vi "db_data_input_b2g_t1_cod_conc.vi"() -> ()   [LabVIEW 2011]
uses:
  <vilib>/Platform/TimedLoop/XDataNode/timing_clust.ctl
  <vilib>/Platform/TimedLoop/XDataNode/nitl_modes.ctl
  <vilib>/Platform/TimedLoop/XDataNode/wakeup.ctl
  <vilib>/addons/database/Connection.llb/DB Tools Open Connec (Path).vi
  <vilib>/Platform/TimedLoop/XDataNode/XDataNode.xnode
  <vilib>/addons/database/_DB Variant To Data/Database Variant To Data.xnode
  <vilib>/Platform/TimedLoop/XDataNode/XDNodeRunTimeDep.lvlib
  <vilib>/addons/database/NI_Database_API.lvlib
panel:
  in  "send data":bool
  in  "COD concentration [mg/l]":u32
  in  "Sampling Timestamp":timestamp format="%<%X\n%x>T"
  in  "Reload":bool
  out "B2G_T1_COD_conc":string[][](table)
  in  "stop":bool
  # "Write COD data of Tank 1 \nto the database"
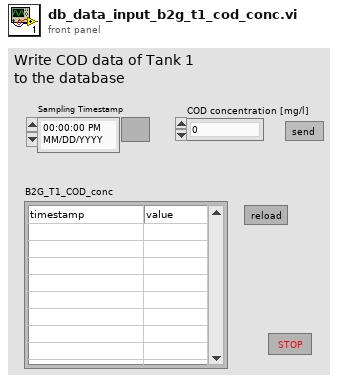
[diagram p1: front panel]
types:
  T1 = typedef "NI_Database_API.lvlib/Conn ObjectReference.ctl" = refnum<k1>
  T2 = typedef "XDNodeRunTimeDep.lvlib/timing_clust.ctl" = cluster{"Expected End [f-1]":u64, "Actual End [f-1]":u64, "Finished Late? [f-1]":bool, "Expected End [i-1]":u64, "Actual End [i-1]":u64, "Finished Late? [i-1]":bool, "Expected Start [i]":u64, "Actual Start [i]":u64, "Expected Start [f]":u64, "Actual Start [f]":u64, "Source Name":string, "Structure Name":string, "Period":i64, "Deadline":i64, "Offset":i64, "Start":i64, "Priority":i32, "Timeout":i32, "Mode":T3, "Wakeup Reason":T4, "Error":errorcluster, "Source Type":string, "Secondary Source Type":string, "Global End Time":u64, "Global Start Time":u64, "Frame Duration":u64, "Iteration Duration":u64, "Assigned CPU":i32, "I/O Scan Engine Mode":u32}
  T3 = typedef "XDNodeRunTimeDep.lvlib/nitl_modes.ctl" = enum32{"No Change", "Process missed periods, maintain original phase", "Discard missed periods, maintain original phase", "Process missed periods, ignore original phase", "Discard missed periods, ignore original phase"}
  T4 = typedef "XDNodeRunTimeDep.lvlib/wakeup.ctl" = enum32{"Normal", "Aborted", "Asynchronous wakeup", "Timing source error", "Timed loop error", "Timeout"}
  T5 = cluster{"Sampling Timestamp":timestamp, "COD concentration [mg/l]":u32}
  T6 = enum32{"invalid app kind", "Development System", "Run Time System", "Student Edition", "Embedded LabVIEW", "Evaluation", "Custom"}
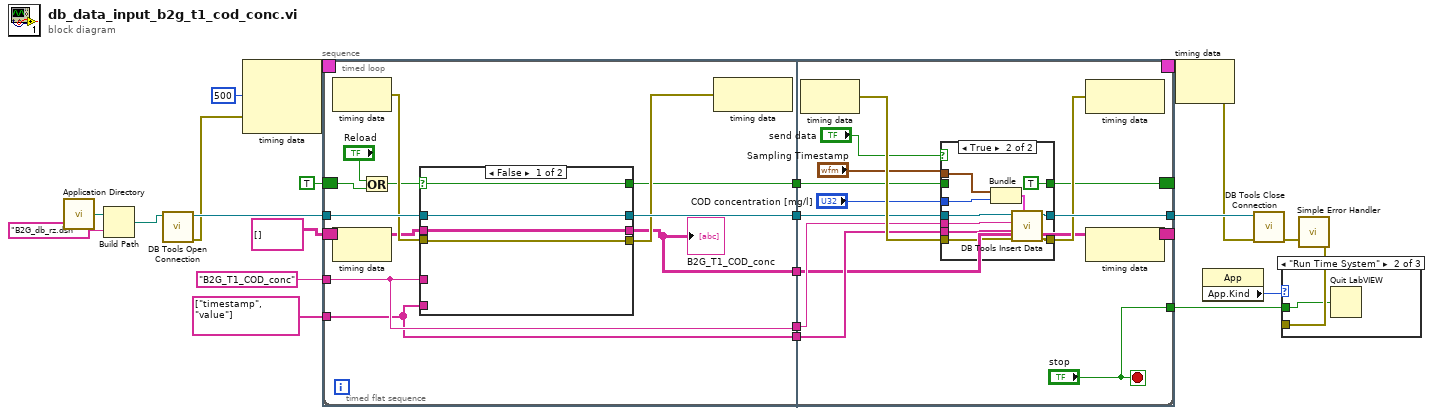
[diagram p0: block diagram]
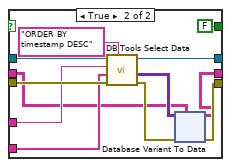
[diagram p4: hidden frame]
diagram:
  n1 = call <vilib>:"Application Directory.vi"() -> ("Application Directory"=w3:path)
  n2 = Build Path(base path=w3, name or relative path="B2G_db_rz.dsn" ("Name of ini file 2")) -> (appended path=w1:path)
  n3 = call-poly <vilib>:"DB Tools Open Connection.vi"("connection information"=w1) -> ("error out"=w13:errorcluster, "connection reference"=w15:T1)  [unwired: 7 in]
  n4 = node-c288(i64 500 ("Period"), w13) -> (w18:T2)  [unwired: 1 in]
  n5 = timed-loop {
    timing: w18 -> [_]
    timing-out: [_] -> w17
    tunnel: w15 -> [w27]
    tunnel: [w26] -> w14
    shift-right: [w25] -> _
    shift-left: TRUE -> [w24]
    tunnel: "B2G_T1_COD_conc" ("table") -> [w23]
    tunnel: string[] ["timestamp", "value"] ("columns") -> [w22]
    tunnel: [w21] -> w7
    shift-right: [w20] -> _
    shift-left: string[][] [] ("data") -> [w19]
    stop <- "stop" stop-if-true
    n6 = timed-sequence {
      timing: _ -> [_]
      timing-out: _ -> [_]
      tunnel: w27 -> [w41]
      tunnel: [w40] -> w26
      tunnel: [w39] -> w25
      tunnel: w24 -> [w38]
      tunnel: w23 -> [w37]
      tunnel: w22 -> [w36]
      tunnel: [w31] -> w21
      tunnel: [w29] -> w20
      tunnel: w19 -> [w28]
      n7 = timed-flat-sequence {
        tunnel: w41 -> [w53]
        tunnel: [w51] -> w35
        tunnel: [w49] -> w34
        tunnel: w38 -> [w48]
        tunnel: w37 -> [w45]
        tunnel: w36 -> [w44]
        tunnel: [w45] -> w33
        tunnel: [w44] -> w32
        tunnel: [w42] -> w30
        tunnel: w28 -> [w46]
        tunnel: [w131] -> w40
        tunnel: w35 -> [w128]
        tunnel: w34 -> [w121]
        tunnel: [w122] -> w39
        tunnel: w33 -> [w127]
        tunnel: w32 -> [w126]
        tunnel: ["stop"] -> w31
        tunnel: w30 -> [w119]
        tunnel: [w119] -> w29
        frame #0 {
          n8 = node-c288() -> (w52:errorcluster)  [unwired: 1 in]
          n9 = Or(x="Reload", y=w48) -> (x .or. y?=w43:bool)
          n10 = case shown="False" w43 {
            selector: w43 -> [w55 _]
            tunnel: w53 -> [w57 w69]
            tunnel: w52 -> [w56 w68]
            tunnel: [w57 w67] -> w51
            tunnel: [w56 w64] -> w50
            tunnel: [w54 w63] -> w42
            tunnel: [w55 FALSE] -> w49
            tunnel: w46 -> [w54 w58]
            tunnel: w45 -> [_ w61]
            tunnel: w44 -> [_ w60]
            frame False {
            }
            frame True {
              n11 = call <vilib>:"DB Tools Select Data.vi"("condition"="ORDER BY timestamp DESC", "error in (no error)"=w68, "columns"=w60, "table"=w61, "connection reference"=w69) -> ("error out"=w65:errorcluster, "data"=w66:variant[][], "connection reference out"=w67:T1)  [unwired: 1 in]
              n12 = xnode "Database Variant To Data"("database variant"=w66, "error in"=w65, "type"=w58) -> ("data"=w63:string[][], "error out"=w64:errorcluster)
            }
          }
          "B2G_T1_COD_conc" <- w42
          n13 = node-c288(w50) -> ()  [unwired: 1 out]
        }
        frame #1 {
          n14 = node-c288() -> (w130:errorcluster)  [unwired: 1 in]
          n15 = case shown="True" "send data" {
            tunnel: [w133 w144] -> w131
            tunnel: w130 -> [w132 w143]
            tunnel: [w132 w142] -> w129
            tunnel: w128 -> [w133 w141]
            tunnel: w127 -> [_ w140]
            tunnel: w126 -> [_ w139]
            tunnel: "Sampling Timestamp" -> [_ w138]
            tunnel: "COD concentration [mg/l]" -> [_ w137]
            tunnel: [w134 TRUE] -> w122
            tunnel: w121 -> [w134 _]
            frame False {
            }
            frame True {
              n16 = Bundle("Sampling Timestamp"=w138, "COD concentration [mg/l]"=w137) -> (w136:T5)  [unwired: 1 in]
              n17 = call <vilib>:"DB Tools Insert Data.vi"("data"=w136, "error in (no error)"=w143, "columns"=w139, "table"=w140, "connection reference"=w141) -> ("error out"=w142:errorcluster, "connection reference out"=w144:T1)  [unwired: 5 in]
            }
          }
          n18 = node-c288(w129) -> ()  [unwired: 1 out]
        }
      }
    }
    n19 = node-c288() -> ()  [unwired: 1 in, 1 out]
    n20 = node-c288() -> ()  [unwired: 1 in, 1 out]
  }
  n21 = node-c288(w17) -> (w12:errorcluster)
  n22 = property class="App"() -> ("App.Kind"=w5:T6)  [unwired: 2 in, 2 out]
  n23 = call <vilib>:"DB Tools Close Connection.vi"("error in (no error)"=w12, "connection reference"=w14) -> ("error out"=w6:errorcluster)  [unwired: 5 in]
  n24 = call <vilib>:"Simple Error Handler.vi"("error in (no error)"=w6) -> ("error out"=w4:errorcluster)  [unwired: 4 in, 4 out]
  n25 = case shown="\"Run Time System\"" w5 {
    tunnel: w7 -> [_ w152 _]
    tunnel: w4 -> [_ _ _]
    frame "invalid app kind", Default {
    }
    frame "Run Time System" {
      n26 = Quit LabVIEW(quit? (T)=w152) -> ()
    }
    frame "Development System" {
    }
  }
